vi "VerifSteps.vi"(8 "error in (no error)":errorcluster, 11 "TelFocus in":refnum<class "TelFocus.lvclass">) -> (0 "error out":errorcluster, 2 "continua?":bool, 3 "TelFocus out":refnum<class "TelFocus.lvclass">)   [LabVIEW 2018, in "TelFocus.lvclass"]
uses:
  TelFocus.lvclass
  TelFocus.lvclass/TelFocus.ctl
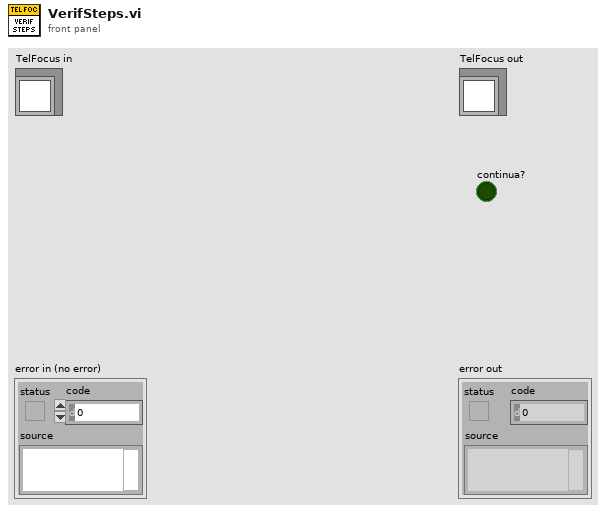
[diagram p1: front panel]
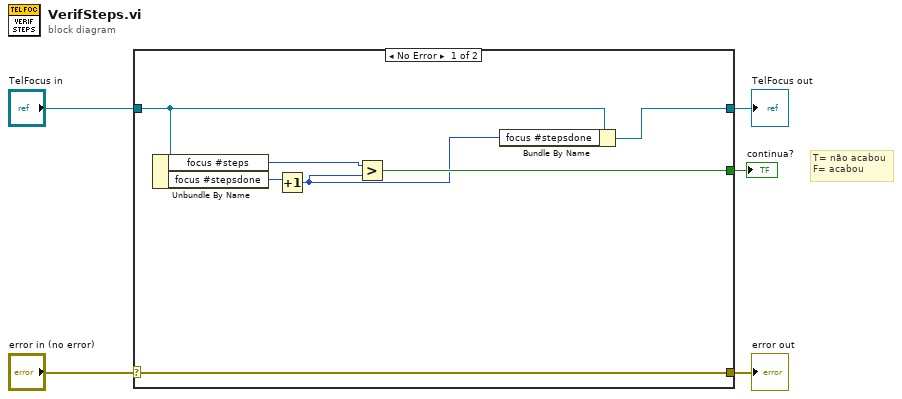
[diagram p0: block diagram]
diagram:
  # "T= não acabou\nF= acabou"
  n1 = case shown="No Error" "error in (no error)" {
    selector: "error in (no error)" -> [w12 w14]
    tunnel: [w12 w14] -> w4
    tunnel: [w6 w13] -> w2
    tunnel: "TelFocus in" -> [w8 w13]
    tunnel: [w9 _] -> w1
    frame No Error {
      n2 = Unbundle By Name(w8) -> ("focus #steps"=w10:u32, "focus #stepsdone"=w11:u32)
      n3 = Increment(x=w11) -> (x+1=w7:u32)
      n4 = Greater?(x=w10, y=w7) -> (0:w9:bool)
      n5 = Bundle By Name(cluster=w8, "focus #stepsdone"=w7) -> (w6:refnum<class "TelFocus.lvclass">)
    }
    frame Error {
    }
  }
  "error out" <- w4
  "TelFocus out" <- w2
  "continua?" <- w1
